vi "sub_Gslam-2.vi"(10 "hz":dbl[][][](array[numeric]), 11 "hxDR":cluster{"x":dbl, "y":dbl, "yaw":dbl}[](array[cluster])) -> ()   [LabVIEW 2019]
uses:
  <vilib>/Analysis/Matrix/Datatypes/RealMatrix.ctl
  Ctrl/cmd_common.ctl
  <vilib>/Analysis/Matrix/Numeric/Conversions/Array To Matrix - RA2.vi
  <vilib>/Analysis/Matrix/Numeric/Conversions/Array To Matrix - RA.vi
  <vilib>/Analysis/Matrix/Numeric/Add/Add - RM,RM.vi
  <vilib>/Analysis/baseanly.llb/Real Inverse Matrix.vi
  <vilib>/Analysis/Matrix/Numeric/Multiply/Multiply - RM,RM.vi
  <vilib>/Analysis/Matrix/NI_Matrix.lvlib
  <vilib>/Analysis/NI_AALBase.lvlib
panel:
  out "A + B 2":T1
  out "submatrix":T1
  out "A + B":T1
  out "H old":T1
  out "Intensity Graph 2":dbl[][](graph)
  out "H new":T1
  out "H inv":T1
  out "dx[i*3:i*3+3,0]":T1
  out "x_dr":cluster{"x":dbl, "y":dbl, "yaw":dbl}
  out "Numeric":i32
  out "i2":i32
  out "error":i32 caption="에러"
  out "-x":T1
  out "i1":i32
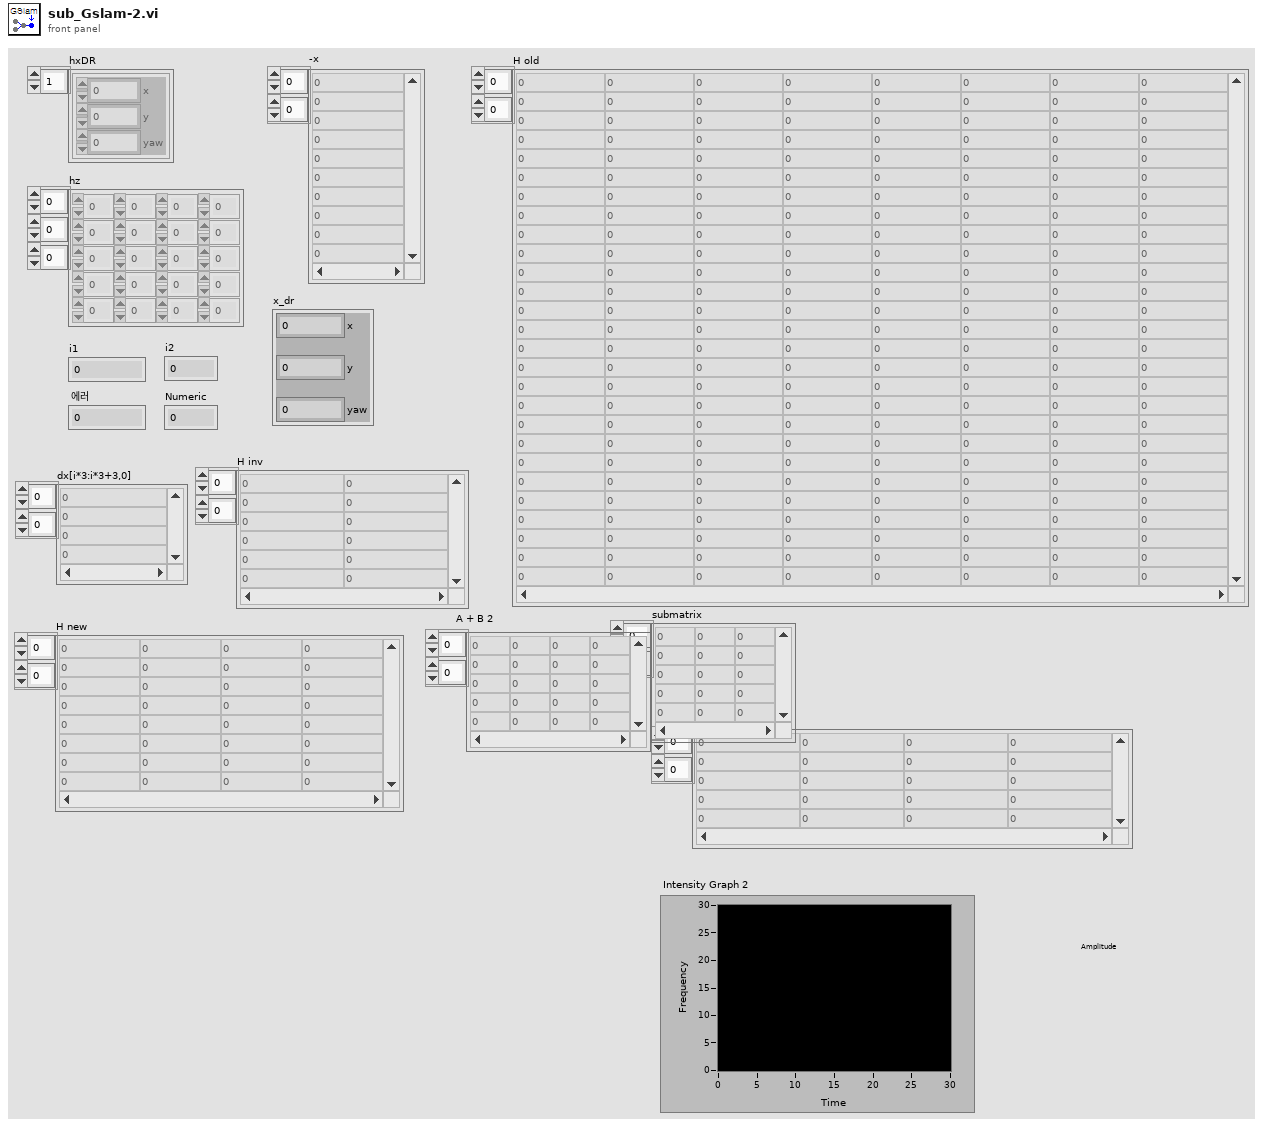
[diagram p1: front panel]
types:
  T1 = typedef "NI_Matrix.lvlib/RealMatrix.ctl" = dbl[][]
  T2 = typedef "cmd_common.ctl" = enum16{"read", "write"}
  T3 = cluster{"Q Sim":T1, "R Sim":T1, "DT":dbl, "SIM_TIME":dbl, "MAX_RANGE":dbl, "STATE_SIZE":i32, "C_SIGMA 1":dbl, "C_SIGMA 2":dbl, "C_SIGMA 3":dbl, "MAX_ITR":u32}
  T4 = cluster{"e":T1, "omega":T1, "d1":dbl, "d2":dbl, "yaw1":dbl, "yaw2":dbl, "angle1":dbl, "angle2":dbl, "id1":i32, "id2":i32}[]
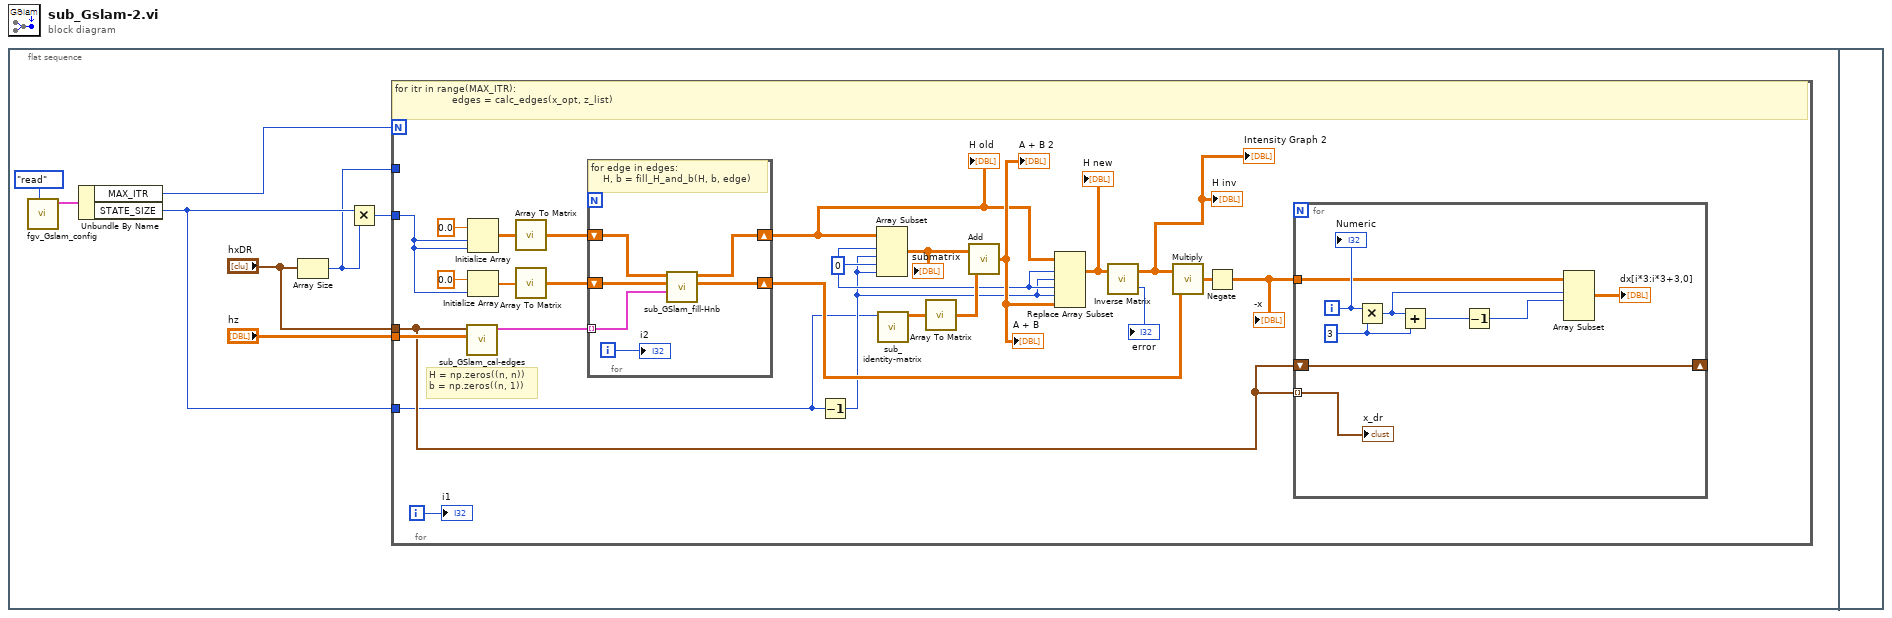
[diagram p0: block diagram]
diagram:
  n1 = flat-sequence {
    frame #0 {
      n2 = call "fgv_Gslam_config.vi"("cmd"=cmd_common."read") -> ("G cofnig out"=w7:T3)  [unwired: 10 in]
      n3 = Unbundle By Name(w7) -> ("MAX_ITR"=w5:u32, "STATE_SIZE"=w2:i32)
      n4 = Array Size(array="hxDR") -> (size(s)=w1:i32)
      n5 = Multiply(x=w2, y=w1) -> (x*y=w4:i32)
      n6 = for {
        N: w5 -> [_]
        tunnel: "hz" -> [w33]
        tunnel: "hxDR" -> [w16]
        tunnel: w4 -> [w29]
        tunnel: w2 -> [w14]
        tunnel: w1 -> [_]
        i -> [w32]
        w19 = 0 ("행 1")
        # "H = np.zeros((n, n))\nb = np.zeros((n, 1))"
        # "for itr in range(MAX_ITR):\n                   edges = calc_edges(x_opt, z_list)"
        n7 = call "sub_GSlam_cal-edges.vi"("z_list"=w33, "x_list"=w16) -> ("edge arr"=w26:T4)  [unwired: 8 in, 1 out]
        n8 = Initialize Array(0.0 ("원소"), w29, w29) -> (w28:dbl[][])
        n9 = Initialize Array(0.0 ("원소"), w29) -> (w27:dbl[])
        n10 = call-poly <vilib>:"Array To Matrix.vi"("Real 2D Array"=w28) -> ("Real Matrix"=w25:T1)
        n11 = call-poly <vilib>:"Array To Matrix.vi"("Real 1D Array"=w27) -> ("Real Matrix (Column Vector)"=w24:T1)
        n12 = for {
          tunnel: w26 -> [w47] mode=indexing
          shift-right: [w46] -> w9
          shift-left: w25 -> [w43]
          shift-right: [w45] -> w17
          shift-left: w24 -> [w48]
          i -> [w44]
          # "for edge in edges:\n    H, b = fill_H_and_b(H, b, edge)"
          n13 = call "sub_GSlam_fill-Hnb.vi"("edge in"=w47, "b"=w48, "H"=w43) -> ("b out"=w45:T1, "H out"=w46:T1)  [unwired: 7 in]
          "i2" <- w44
        }
        "H old" <- w9
        n14 = Decrement(x=w14) -> (x-1=w15:i32)
        n15 = Array Subset(array=w9, index (row)=w19, length (row)=w15, index (col)=w19, length (col)=w15) -> (w23:T1)
        "submatrix" <- w23
        n16 = call "sub_identity-matrix.vi"("STATE_SIZE"=w14) -> ("identity"=w22:dbl[][])  [unwired: 10 in]
        n17 = call-poly <vilib>:"Array To Matrix.vi"("Real 2D Array"=w22) -> ("Real Matrix"=w21:T1)
        n18 = call-poly <vilib>:"Add.vi"("Real Matrix B"=w21, "Real Matrix A"=w23) -> ("A + B"=w20:T1)
        "A + B" <- w20
        "A + B 2" <- w20
        n19 = Replace Array Subset(array=w9, new element=w20, index (dim 0)=w19, index (dim 1)=w15, index (dim 2)=w19, index (dim 3)=w15) -> (w11:T1)
        "H new" <- w11
        n20 = call-poly <vilib>:"Inverse Matrix.vi"("Input Matrix"=w11) -> ("error"=→"error":i32, "Inverse Matrix"=w10:T1)  [unwired: 1 in]
        "H inv" <- w10
        "Intensity Graph 2" <- w10
        n21 = call-poly <vilib>:"Multiply.vi"("Real Matrix B"=w17, "Real Matrix A"=w10) -> ("A * B"=w18:T1)
        n22 = Negate(x=w18) -> (-x=w12:T1)
        "-x" <- w12
        n23 = for {
          shift-right: [w40] -> _
          shift-left: w16 -> [w40]
          tunnel: w16 -> [w39] mode=indexing
          tunnel: w12 -> [w38]
          i -> [w42]
          w41 = 3 ("y")
          n24 = Multiply(x=w42, y=w41) -> (x*y=w37:i32)
          n25 = Add(x=w37, y=w41) -> (x+y=w36:i32)
          n26 = Decrement(x=w36) -> (x-1=w34:i32)
          n27 = Array Subset(array=w38, index (row)=w37, length (row)=w34) -> (→"dx[i*3:i*3+3,0]":T1)  [unwired: 2 in]
          "Numeric" <- w42
          "x_dr" <- w39
        }
        "i1" <- w32
      }
    }
    frame #1 {
    }
  }
